vi "Process Data.vi"(7 "AdasLvTemplate in":refnum<class "AdasLvTemplate.lvclass">, 8 "error in":errorcluster, 11 "Node in":refnum<class "BLS Climate Chamber Template.lvclass">) -> (0 "error out":errorcluster, 3 "Node out":refnum<class "BLS Climate Chamber Template.lvclass">, 5 "AdasLvTemplate out":refnum<class "AdasLvTemplate.lvclass">)   [LabVIEW 2023, in "BLS Climate Chamber Template.lvlib" / "BLS Climate Chamber Template.lvclass"]
uses:
  BLS Climate Chamber Template.lvclass
  BLS Climate Chamber Template.lvclass/BLS Climate Chamber Template.ctl
  C:/Program Files/National Instruments/BLS plugin/Capabilities/Capabilities/High Level Capabilities/Climate Chamber/Climate Chamber.lvclass
  C:/Program Files/National Instruments/BLS plugin/Capabilities/Capabilities/High Level Capabilities/Climate Chamber/Humidity Grad Read Single.vi
  C:/Program Files/National Instruments/BLS plugin/Capabilities/Capabilities/High Level Capabilities/Climate Chamber/Humidity Read Single.vi
  C:/Program Files/National Instruments/BLS plugin/Capabilities/Capabilities/High Level Capabilities/Climate Chamber/Humidity Max Read Single.vi
  C:/Program Files/National Instruments/BLS plugin/Capabilities/Capabilities/High Level Capabilities/Climate Chamber/Humidity Min Read Single.vi
  C:/Program Files/National Instruments/BLS plugin/Capabilities/Capabilities/High Level Capabilities/Climate Chamber/Humidity Write Single.vi
  C:/Program Files/National Instruments/BLS plugin/Capabilities/Capabilities/High Level Capabilities/Climate Chamber/Temperature Grad Read Single.vi
  C:/Program Files/National Instruments/BLS plugin/Capabilities/Capabilities/High Level Capabilities/Climate Chamber/Temperature Max Read Single.vi
  C:/Program Files/National Instruments/BLS plugin/Capabilities/Capabilities/High Level Capabilities/Climate Chamber/Temperature Min Read Single.vi
  C:/Program Files/National Instruments/BLS plugin/Capabilities/Capabilities/High Level Capabilities/Climate Chamber/Temperature Write Single.vi
  C:/Program Files/National Instruments/BLS plugin/Capabilities/Capabilities/High Level Capabilities/Climate Chamber/Temperature Read Single.vi
  <vilib>/ADAS Replay HIL/ADAS Plugin Utilities/AdasLvTemplate/AdasLvTemplate.lvclass
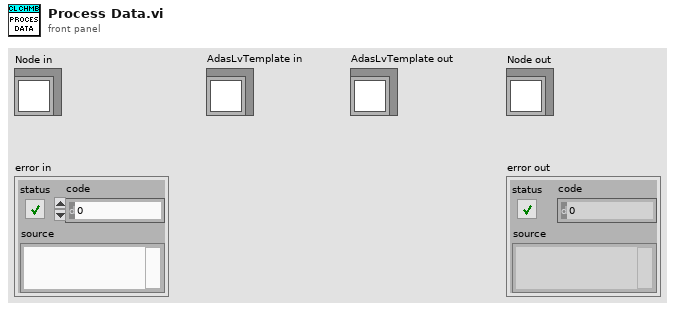
[diagram p1: front panel]
types:
  T1 = typedef "BLS Climate Chamber Template.lvlib/BLS Climate Chamber Template.lvclass/Configuration Params.ctl" = cluster{"Common":T2, "Amount of Channels":u32, "Address":string}
  T2 = typedef "Template Node.lvlib/Template Node.lvclass/Common Configuration Params.ctl" = cluster{"Iteration Interval (s)":dbl, "T0 (ns)":u64, "Priority":i32, "Processor":i32, "Wait in Ready State":bool}
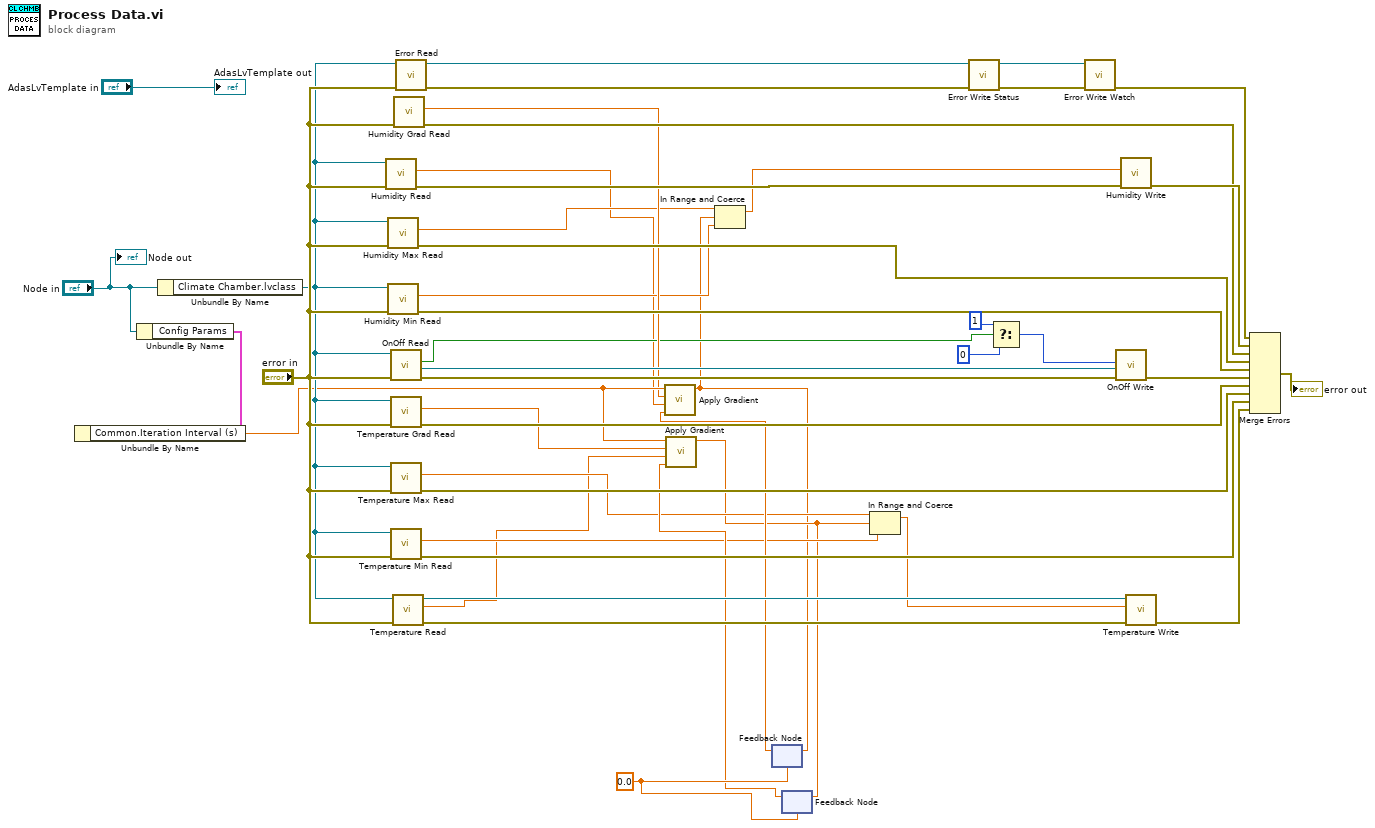
[diagram p0: block diagram]
diagram:
  w16 = 0.0 ("Current Setpoint")
  n1 = Unbundle By Name("Node in") -> ("Config Params"=w22:T1)
  n2 = Unbundle By Name(w22) -> ("Common.Iteration Interval (s)"=w20:dbl)
  n3 = Unbundle By Name("Node in") -> ("Climate Chamber.lvclass"=w37:refnum<class "Climate Chamber.lvclass">)
  n4 = call-poly "Humidity Read.vi"("error in"="error in", "Climate Chamber in"=w37) -> ("error out"=w39:errorcluster, "Humidity SP"=w8:dbl)  [unwired: 6 in, 2 out]
  n5 = call-poly "Humidity Max Read.vi"("error in"="error in", "Climate Chamber in"=w37) -> ("error out"=w29:errorcluster, "Humidity Max SP"=w10:dbl)  [unwired: 6 in, 2 out]
  n6 = call-poly "Humidity Min Read.vi"("error in"="error in", "Climate Chamber in"=w37) -> ("error out"=w28:errorcluster, "Humidity Min SP"=w9:dbl)  [unwired: 6 in, 2 out]
  n7 = call "OnOff Read.vi"("error in"="error in", "Climate Chamber in"=w37) -> ("error out"=w43:errorcluster, "OnOff ACT"=w12:bool, "Climate Chamber out"=w38:refnum<class "Climate Chamber.lvclass">)  [unwired: 6 in, 1 out]
  n8 = call-poly "Temperature Grad Read.vi"("error in"="error in", "Climate Chamber in"=w37) -> ("error out"=w26:errorcluster, "Temperature SP"=w18:dbl)  [unwired: 6 in, 2 out]
  n9 = call-poly "Temperature Max Read.vi"("error in"="error in", "Climate Chamber in"=w37) -> ("error out"=w25:errorcluster, "Temperature Max SP"=w6:dbl)  [unwired: 6 in, 2 out]
  n10 = call-poly "Temperature Min Read.vi"("error in"="error in", "Climate Chamber in"=w37) -> ("error out"=w24:errorcluster, "Temperature Min SP"=w5:dbl)  [unwired: 6 in, 2 out]
  n11 = call-poly "Temperature Read.vi"("error in"="error in", "Climate Chamber in"=w37) -> ("error out"=w45:errorcluster, "Temperature SP"=w4:dbl, "Climate Chamber out"=w44:refnum<class "Climate Chamber.lvclass">)  [unwired: 6 in, 1 out]
  n12 = call-poly "Humidity Grad Read.vi"("error in"="error in") -> ("error out"=w30:errorcluster, "Humidity SP"=w19:dbl)  [unwired: 7 in, 2 out]
  n13 = call "Error Read.vi"("error in"="error in", "Climate Chamber in"=w37) -> ("error out"=w41:errorcluster, "Climate Chamber out"=w36:refnum<class "Climate Chamber.lvclass">)  [unwired: 6 in, 2 out]
  n14 = feedback #1(w16) -> (w17:dbl)
  n15 = call "Apply Gradient.vi"("Reminder"=w17, "Setpoint"=w8, "Gradient"=w19, "Iteration Interval"=w20) -> ("Current Setpoint"=w1:dbl)  [unwired: 7 in]
  n16 = In Range and Coerce(upper limit=w10, x=w1, lower limit=w9) -> (coerced(x)=w7:dbl)  [unwired: 1 out]
  n17 = feedback-in #1(w1) -> ()
  n18 = feedback #2(w16) -> (w15:dbl)
  n19 = call "Apply Gradient.vi"("Reminder"=w15, "Setpoint"=w4, "Gradient"=w18, "Iteration Interval"=w20) -> ("Current Setpoint"=w3:dbl)  [unwired: 7 in]
  n20 = feedback-in #2(w3) -> ()
  n21 = In Range and Coerce(upper limit=w6, x=w3, lower limit=w5) -> (coerced(x)=w2:dbl)  [unwired: 1 out]
  n22 = call "Error Write Status.vi"("error in"=w41, "Climate Chamber in"=w36) -> ("error out"=w40:errorcluster, "Climate Chamber out"=w35:refnum<class "Climate Chamber.lvclass">)  [unwired: 8 in]
  n23 = Select(t=1, s=w12, f=0) -> (s? t:f=w11:i32)
  n24 = call "Error Write Watch.vi"("error in"=w40, "Climate Chamber in"=w35) -> ("error out"=w32:errorcluster)  [unwired: 8 in, 1 out]
  n25 = call "OnOff Write.vi"("error in"=w43, "OnOff STS"=w11, "Climate Chamber in"=w38) -> ("error out"=w27:errorcluster)  [unwired: 7 in, 1 out]
  n26 = call-poly "Humidity Write.vi"("error in"=w39, "Humidity AV"=w7) -> ("error out"=w31:errorcluster)  [unwired: 8 in, 1 out]
  n27 = call-poly "Temperature Write.vi"("error in"=w45, "Temperature AV"=w2, "Climate Chamber in"=w44) -> ("error out"=w23:errorcluster)  [unwired: 7 in, 1 out]
  n28 = Merge Errors(w32, w31, w30, w29, w28, w27, w26, w25, w24, w23) -> (→"error out":errorcluster)
  "Node out" <- "Node in"
  "AdasLvTemplate out" <- "AdasLvTemplate in"
